vi "SetAPSxParameter.vi"(8 "error in (no error)":errorcluster caption="错误输入（无错误）", 9 "Param2":i32, 10 "Param1":T1(ring), 11 "hASIC":i32) -> (0 "error out":errorcluster caption="错误输出", 2 "Message":string, 3 "hASIC out":i32)   [LabVIEW 2020]
doc: "该模板用于创建子VI。"
uses:
  APSx.dll/APSx.dll
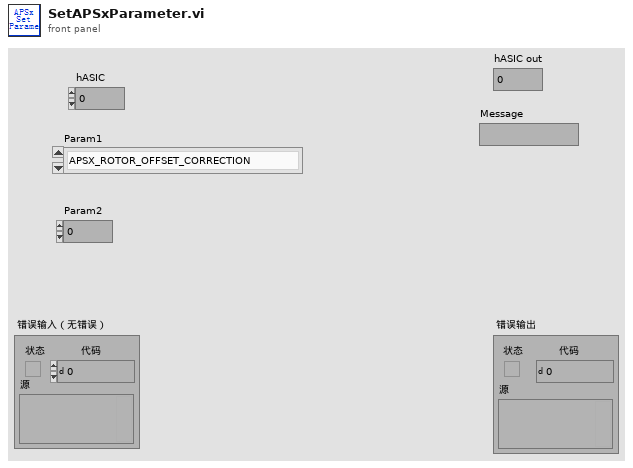
[diagram p1: front panel]
types:
  T1 = enum16{"APSX_ROTOR_OFFSET_CORRECTION", "APSX_SCALING"}
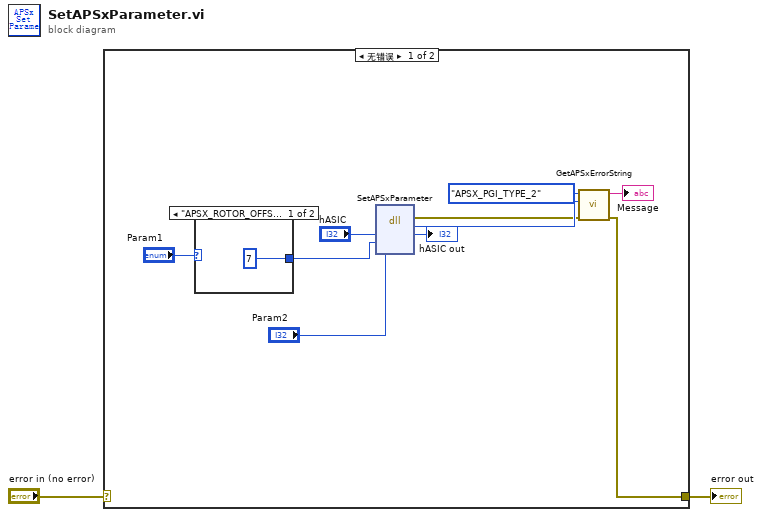
[diagram p0: block diagram]
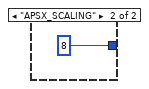
[diagram p2: hidden frame]
diagram:
  n1 = case shown="无错误" "error in (no error)" {
    selector: "error in (no error)" -> [_ w15]
    tunnel: [w4 w15] -> w1
    frame No Error {
      n2 = case shown="\"APSX_ROTOR_OFFSET_CORRECTION\", 默认" "Param1" {
        tunnel: [7 8] -> w9
        frame "APSX_ROTOR_OFFSET_CORRECTION", Default {
        }
        frame "APSX_SCALING" {
        }
      }
      n3 = dll-call lib="PTH2Oabs D程序临时修改280传感器对中台SourcesAPSx.dllAPSx.dll" fn="SetAPSxParameter"("hASIC"="hASIC", "Param1"=w9, "Param2"="Param2") -> (error out=w5:errorcluster, "Code"=w6:i32, "hASIC"=→"hASIC out":i32)  [unwired: 5 in, 1 out]
      n4 = call "GetAPSxErrorString.vi"("error in (no error)"=w5, "ErrorCode"=w6, "PGIType"=enum16{"APSX_PGI_TYPE_1", "APSX_PGI_TYPE_2"}."APSX_PGI_TYPE_2") -> ("error out"=w4:errorcluster, "Message"=→"Message":string)  [unwired: 7 in]
    }
    frame Error {
    }
  }
  "error out" <- w1
